vi "Triggerer.vi"   [LabVIEW 2012]
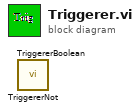
[diagram p0: block diagram]
diagram:
  n1 = call "TriggererNot.vi"() -> ()  [unwired: 10 in, 2 out]
  n2 = call "TriggererBoolean.vi"() -> ()  [unwired: 10 in, 2 out]
